vi "Log String.vi"(1 "Message":string) -> (0 "Log String":string)   [LabVIEW 2017]
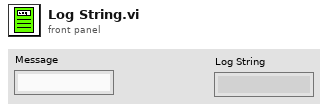
[diagram p1: front panel]
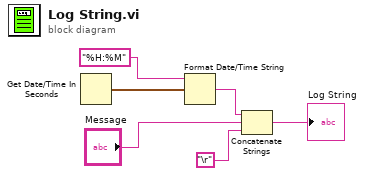
[diagram p0: block diagram]
diagram:
  n1 = Get Date/Time In Seconds() -> (seconds since 1Jan1904=w5:timestamp)
  n2 = Format Date/Time String(time format string (%c)="%H:%M", seconds (now)=w5) -> (date/time string=w6:string)  [unwired: 1 in]
  n3 = Concatenate Strings(w6, "Message", "\r") -> (→"Log String":string)
